vi "pdNormalize_IV.vi"(0 "405 Data":T2, 5 "532 Data":T3, 7 "660 Data":T4, 9 "785 Data":T1, 11 "785 PD Cal":dbl, 12 "405 PD Cal":dbl, 13 "532 PD Cal":dbl, 14 "660 PD Cal":dbl) -> (4 "Output Cluster":cluster{dbl, dbl, dbl, dbl}, 6 "405 New Array":dbl[](array[numeric]), 8 "532 New Array":dbl[](array[numeric]), 10 "660 New Array":dbl[](array[numeric]), 15 "785 New Array":dbl[](array[numeric]))   [LabVIEW 2011]
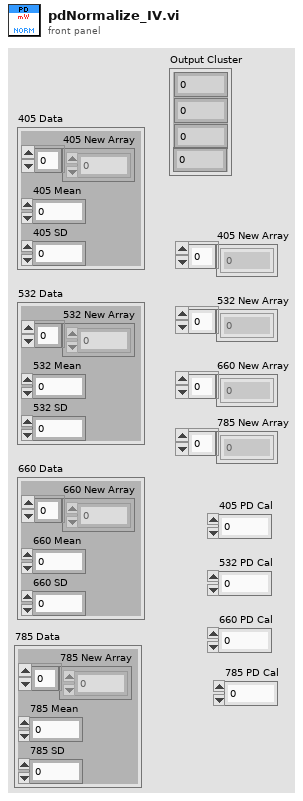
[diagram p1: front panel]
types:
  T1 = cluster{"785 New Array":dbl[], "785 Mean":dbl, "785 SD":dbl}
  T2 = cluster{"405 New Array":dbl[], "405 Mean":dbl, "405 SD":dbl}
  T3 = cluster{"532 New Array":dbl[], "532 Mean":dbl, "532 SD":dbl}
  T4 = cluster{"660 New Array":dbl[], "660 Mean":dbl, "660 SD":dbl}
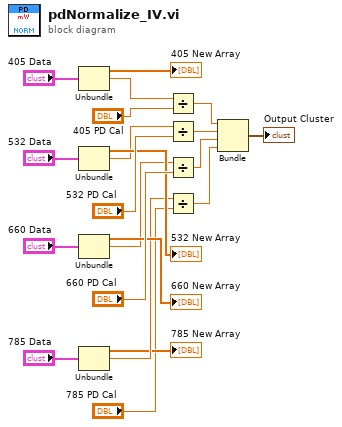
[diagram p0: block diagram]
diagram:
  n1 = Unbundle("405 Data") -> ("405 New Array"=→"405 New Array":dbl[], "405 Mean"=w8:dbl)  [unwired: 1 out]
  n2 = Unbundle("532 Data") -> ("532 New Array"=→"532 New Array":dbl[], "532 Mean"=w10:dbl)  [unwired: 1 out]
  n3 = Unbundle("660 Data") -> ("660 New Array"=→"660 New Array":dbl[], "660 Mean"=w11:dbl)  [unwired: 1 out]
  n4 = Unbundle("785 Data") -> ("785 New Array"=→"785 New Array":dbl[], "785 Mean"=w5:dbl)  [unwired: 1 out]
  n5 = Divide(x=w8, y="405 PD Cal") -> (x/y=w2:dbl)
  n6 = Divide(x=w10, y="532 PD Cal") -> (x/y=w9:dbl)
  n7 = Divide(x=w11, y="660 PD Cal") -> (x/y=w1:dbl)
  n8 = Divide(x=w5, y="785 PD Cal") -> (x/y=w6:dbl)
  n9 = Bundle(w2, w9, w1, w6) -> (→"Output Cluster":cluster{dbl, dbl, dbl, dbl})  [unwired: 1 in]
